vi "7.1 Complex Situation.vi"() -> ()   [LabVIEW 2017]
uses:
  3a5d3adc-f18e-4b24-90ad-4b548b3d9b49.vi
  86d59eec-a28c-42d3-be80-1aa62744661d.vi
  addons/API-String-Arugments-Support/_Support/Convert API String Arguments to Data(variant).vi
  8b979ef5-f5f6-4d36-b0d8-cf42d7dfdfe2.vi
  0333efe5-f0fb-4901-b6dd-db031cec30c6.vi
panel:
  out "Retrieve Array 2":T1={"Empty API String"="", "1D DBL"=[3.12, 4.11, 5.0], "Retrieved Data"=[3.12, 4.11, 5.0]}
  out "Retrieve Array 1":T1={"Empty API String"="", "1D DBL"=[3.12, 4.11, 5.0], "Retrieved Data"=[3.12, 4.11, 5.0]}
  out "Retrieve Cluster Array and keep both Type and default value":T2={"String"=["{BoolArray:[0,1,0,1;1,0,1,0;0,1,0,1];Cluster.Boolean:True}", "BoolArray:[TRUE,FALSE,TRUE,FALSE;FALSE,TRUE,FALSE,TRUE;TRUE,FALSE,TRUE,FALSE];Cluster.Boolean:off"], "Reference Cluster Array"=[{"String"="abc", "BoolArray"=[[TRUE, FALSE, TRUE, FALSE], [FALSE, TRUE, FALSE, TRUE], [TRUE, FALSE, TRUE, FALSE]], "Cluster"={"Boolean"=FALSE}}, {"String"="def", "BoolArray"=[[FALSE, TRUE, FALSE, TRUE], [TRUE, FALSE, TRUE, FALSE], [FALSE, TRUE, FALSE, TRUE]], "Cluster"={"Boolean"=TRUE}}], "Retrieved Cluster Array"=[{"String"="abc", "BoolArray"=[[FALSE, TRUE, FALSE, TRUE], [TRUE, FALSE, TRUE, FALSE], [FALSE, TRUE, FALSE, TRUE]], "Cluster"={"Boolean"=TRUE}}, {"String"="def", "BoolArray"=[[TRUE, FALSE, TRUE, FALSE], [FALSE, TRUE, FALSE, TRUE], [TRUE, FALSE, TRUE, FALSE]], "Cluster"={"Boolean"=FALSE}}]}
  out "Retrieve Cluster Array and keep Type Only":T3={"String"="[{BoolArray:[0,1,0,1;1,0,1,0;0,1,0,1];Cluster.Boolean:True},{BoolArray:[TRUE,FALSE,TRUE,FALSE;FALSE,TRUE,FALSE,TRUE;TRUE,FALSE,TRUE,FALSE];Cluster.Boolean:off}]", "Reference Cluster Array"=[{"String"="abc", "BoolArray"=[[TRUE, FALSE, TRUE, FALSE], [FALSE, TRUE, FALSE, TRUE], [TRUE, FALSE, TRUE, FALSE]], "Cluster"={"Boolean"=FALSE}}, {"String"="def", "BoolArray"=[[FALSE, TRUE, FALSE, TRUE], [TRUE, FALSE, TRUE, FALSE], [FALSE, TRUE, FALSE, TRUE]], "Cluster"={"Boolean"=TRUE}}], "Retrieved Cluster Array"=[{"String"="", "BoolArray"=[[FALSE, TRUE, FALSE, TRUE], [TRUE, FALSE, TRUE, FALSE], [FALSE, TRUE, FALSE, TRUE]], "Cluster"={"Boolean"=TRUE}}, {"String"="", "BoolArray"=[[TRUE, FALSE, TRUE, FALSE], [FALSE, TRUE, FALSE, TRUE], [TRUE, FALSE, TRUE, FALSE]], "Cluster"={"Boolean"=FALSE}}]}
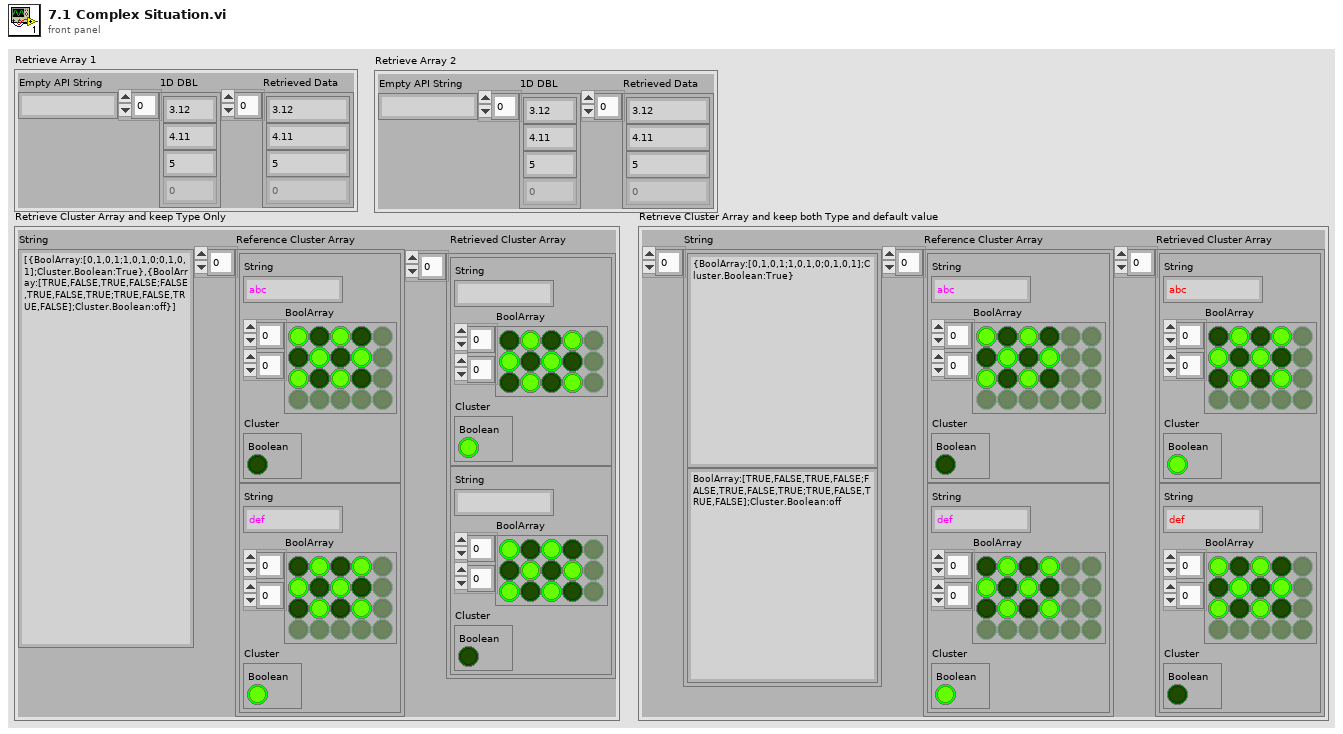
[diagram p1: front panel]
types:
  T1 = cluster{"Empty API String":string, "1D DBL":dbl[], "Retrieved Data":dbl[]}
  T2 = cluster{"String":string[], "Reference Cluster Array":cluster{"String":string, "BoolArray":bool[][], "Cluster":cluster{"Boolean":bool}}[], "Retrieved Cluster Array":cluster{"String":string, "BoolArray":bool[][], "Cluster":cluster{"Boolean":bool}}[]}
  T3 = cluster{"String":string, "Reference Cluster Array":cluster{"String":string, "BoolArray":bool[][], "Cluster":cluster{"Boolean":bool}}[], "Retrieved Cluster Array":cluster{"String":string, "BoolArray":bool[][], "Cluster":cluster{"Boolean":bool}}[]}
  T4 = cluster{"String":string, "BoolArray":bool[][], "Cluster":cluster{"Boolean":bool}}[]
  T5 = cluster{"String":string, "Cluster":cluster{"String":string, "BoolArray":bool[][], "Cluster":cluster{"Boolean":bool}}[], "Data":cluster{"String":string, "BoolArray":bool[][], "Cluster":cluster{"Boolean":bool}}[]}
  T6 = cluster{"String":string, "Data 4":dbl[], "Data":dbl[]}
  T7 = cluster{"String":string, "BoolArray":bool[][], "Cluster":cluster{"Boolean":bool}}
  T8 = cluster{"String":string[], "Cluster":cluster{"String":string, "BoolArray":bool[][], "Cluster":cluster{"Boolean":bool}}[], cluster{"String":string, "BoolArray":bool[][], "Cluster":cluster{"Boolean":bool}}[]}
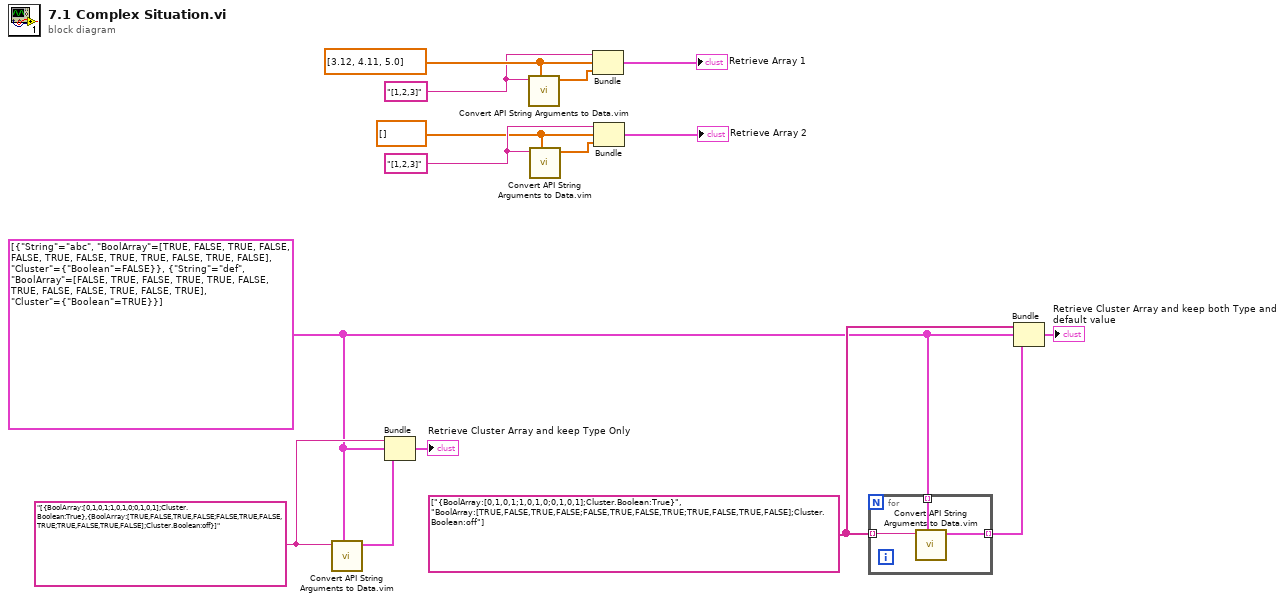
[diagram p0: block diagram]
diagram:
  w4 = "[1,2,3]" ("String")
  w2 = dbl[] [] ("Data 4")
  w5 = "[1,2,3]" ("String")
  w7 = dbl[] [3.12, 4.11, 5.0] ("Data 4")
  w12 = string[] ["{BoolArray:[0,1,0,1;1,0,1,0;0,1,0,1];Cluster.Boolean:True}", "BoolArray:[TRUE,FALSE,TRUE,FALSE;FALSE,TRUE,FALSE,TRUE;TRUE,FALSE,TRUE,FALSE];Cluster.Boolean:off"] ("String")
  w13 = "[{BoolArray:[0,1,0,1;1,0,1,0;0,1,0,1];Cluster.Boolean:True},{BoolArray:[TRUE,FALSE,TRUE,FALSE;FALSE,TRUE,FALSE,TRUE;TRUE,FALSE,TRUE,FALSE];Cluster.Boolean:off}]" ("String")
  w11 = T4 [{"String"="abc", "BoolArray"=[[TRUE, FALSE, TRUE, FALSE], [FALSE, TRUE, FALSE, TRUE], [TRUE, FALSE, TRUE, FALSE]], "Cluster"={"Boolean"=FALSE}}, {"String"="def", "BoolArray"=[[FALSE, TRUE, FALSE, TRUE], [TRUE, FALSE, TRUE, FALSE], [FALSE, TRUE, FALSE, TRUE]], "Cluster"={"Boolean"=TRUE}}] ("Cluster")
  n1 = call "Convert API String Arguments to Data.vim"("Type"=w11, "String"=w13) -> ("Data"=w15:T4)  [unwired: 6 in, 1 out]
  n2 = Bundle("String"=w13, "Cluster"=w11, "Data"=w15) -> (→"Retrieve Cluster Array and keep Type Only":T5)  [unwired: 1 in]
  n3 = call "Convert API String Arguments to Data.vim"("Type"=w7, "String"=w5) -> ("Data"=w8:dbl[])  [unwired: 6 in, 1 out]
  n4 = call "Convert API String Arguments to Data.vim"("Type"=w2, "String"=w4) -> ("Data"=w1:dbl[])  [unwired: 6 in, 1 out]
  n5 = Bundle("String"=w5, "Data 4"=w7, "Data"=w8) -> (→"Retrieve Array 1":T6)  [unwired: 1 in]
  n6 = Bundle("String"=w4, "Data 4"=w2, "Data"=w1) -> (→"Retrieve Array 2":T6)  [unwired: 1 in]
  n7 = for {
    tunnel: w11 -> [w18] mode=indexing
    tunnel: w12 -> [w17] mode=indexing
    tunnel: [w16] -> w10 mode=indexing
    n8 = call "Convert API String Arguments to Data.vim"("Type"=w18, "String"=w17) -> ("Data"=w16:T7)  [unwired: 6 in, 1 out]
  }
  n9 = Bundle("String"=w12, "Cluster"=w11, w10) -> (→"Retrieve Cluster Array and keep both Type and default value":T8)  [unwired: 1 in]
